vi "agilent_34970A_initialize.vi"(3 "resistance channels (csv)":string, 4 "voltage channels (csv)":string, 5 "Agilent 34970A Port":refnum<visa-resource-name>="COM35") -> (0 "Error Message":string="+0,\"No error\"\r\n", 1 "34970A Error Out":errorcluster={"status"=FALSE, "code"=-1074001665, "source"="HP34970A Error Query;\ninstrument reports:\n+0,\"No error\"\r\n"}, 2 "34970A Port Out":refnum<visa-resource-name>="COM35")   [LabVIEW 2010]
panel:
  in  "Resistance Advanced Config":T1={"Offset Compensation (F:Off)"=FALSE, "Aperture Value (.4)"=0.4, "Aperture (1:Minimum)"=1, "NPLC (1)"=2, "Integration Time (F:Aperture)"=TRUE} {"NPLC (1)" items=[".02", ".2", "1", "2", "10", "20", "100", "200", "Minimum", "Maximum"]; "Aperture (1:Minimum)" items=["Manual", "Minimum", "Maximum"]; "Aperture Value (.4)" min=0.4 max=4.0 format="%.2f"}
  in  "Voltage Advanced Config":T2={"Aperture Value (.4)"=0.4, "Aperture (1:Minimum)"=1, "NPLC (1)"=2, "Bandwidth (3 Hz)"=0, "Input Impedance (F:Fixed)"=FALSE, "Integration Time (F:Aperture)"=TRUE} {"Bandwidth (3 Hz)" items=["3 Hz", "20 Hz", "200 Hz", "Minimum", "Maximum"]; "NPLC (1)" items=[".02", ".2", "1", "2", "10", "20", "100", "200", "Minimum", "Maximum"]; "Aperture (1:Minimum)" items=["Manual", "Minimum", "Maximum"]; "Aperture Value (.4)" min=0.4 max=4.0 format="%.2f"}
  in  "Serial Port Configuration":T3={"Timeout Value (10000)"=10000, "Baud Rate (57600)"=enum."57600", "Flow Control (1:XON/XOFF)"=enum."XON / XOFF"}
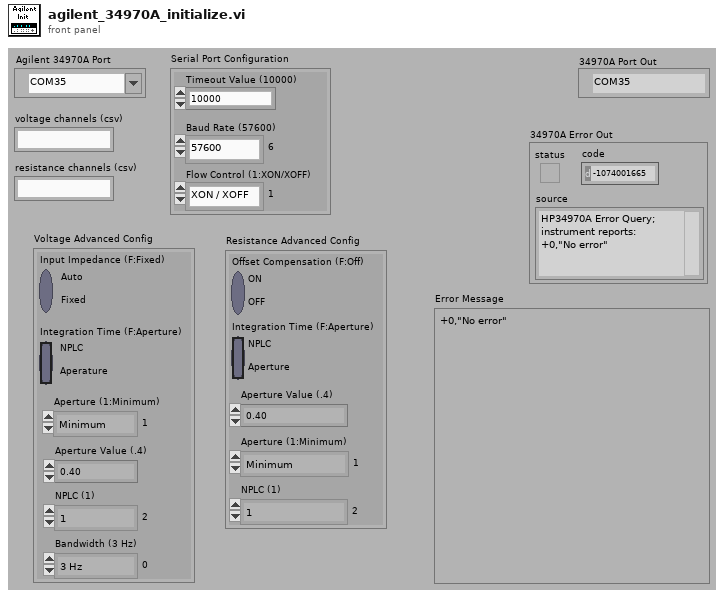
[diagram p1: front panel]
types:
  T1 = cluster{"Offset Compensation (F:Off)":bool, "Aperture Value (.4)":dbl, "Aperture (1:Minimum)":u16, "NPLC (1)":u16, "Integration Time (F:Aperture)":bool}
  T2 = cluster{"Aperture Value (.4)":dbl, "Aperture (1:Minimum)":u16, "NPLC (1)":u16, "Bandwidth (3 Hz)":u16, "Input Impedance (F:Fixed)":bool, "Integration Time (F:Aperture)":bool}
  T3 = cluster{"Timeout Value (10000)":u32, "Baud Rate (57600)":enum16{"1200", "2400", "4800", "9600", "19200", "38400", "57600", "115200"}, "Flow Control (1:XON/XOFF)":enum16{"None", "XON / XOFF", "RTS / CTS", "DTR / DSR"}}
  T4 = enum16{"100 Ohm", "1 kOhm", "10 kOhm", "100 kOhm", "1 MOhm", "10 MOhm", "100 MOhm", "Minimum", "Maximum"}
  T5 = enum16{"100 mV", "1 V", "10 V", "100 V", "300 V", "Minimum", "Maximum"}
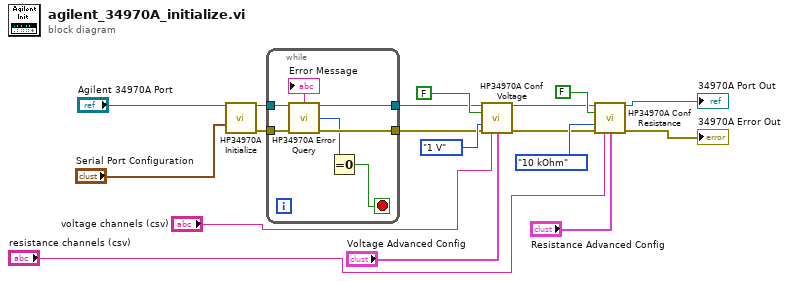
[diagram p0: block diagram]
diagram:
  n1 = call "HP34970A Initialize.vi"("VISA resource name"="Agilent 34970A Port", "Serial Port Configuration"="Serial Port Configuration") -> ("VISA resource name out"=w16:refnum<visa-resource-name>, "error out"=w15:errorcluster)  [unwired: 12 in]
  n2 = while {
    tunnel: w16 -> [w25]
    tunnel: w15 -> [w24]
    tunnel: [w23] -> w12
    tunnel: [w22] -> w11
    stop <- w19 stop-if-true
    n3 = call "HP34970A Error Query.vi"("VISA resource name"=w25, "error in (no error)"=w24) -> ("VISA resource name out"=w23:refnum<visa-resource-name>, "Error"=w20:i32, "Error Message"=→"Error Message":string, "error out"=w22:errorcluster)  [unwired: 10 in]
    n4 = Equal To 0?(x=w20) -> (x = 0?=w19:bool)
  }
  n5 = call "HP34970A Conf Voltage.vi"("VISA resource name"=w12, "AC/DC (F:DC)"=FALSE, "Range (6:Max)"=T5."1 V", "error in (no error)"=w11, "Channel List (empty)"="voltage channels (csv)", "Advanced Config"="Voltage Advanced Config") -> ("VISA resource name out"=w8:refnum<visa-resource-name>, "error out"=w7:errorcluster)  [unwired: 7 in, 1 out]
  n6 = call "HP34970A Conf Resistance.vi"("VISA resource name"=w8, "4 Wire/2 Wire (F:2)"=FALSE ("AC/DC (F:DC)"), "Range (8:Maximum)"=T4."10 kOhm", "error in (no error)"=w7, "Channel List (empty)"="resistance channels (csv)", "Advanced Config"="Resistance Advanced Config") -> ("VISA resource name out"=→"34970A Port Out":refnum<visa-resource-name>, "error out"=→"34970A Error Out":errorcluster)  [unwired: 7 in, 1 out]
